vi "HandleError.vi"(8 "error in (no error)":errorcluster, 11 "Queue in":refnum<queue>) -> (0 "error out":errorcluster, 3 "queue out":refnum<queue>)   [LabVIEW 2019, in "AutoMode.lvlib"]
uses:
  AutoMode.lvlib
  Cluster - AutoModeMessage.ctl
  Enum - AutoModeState.ctl
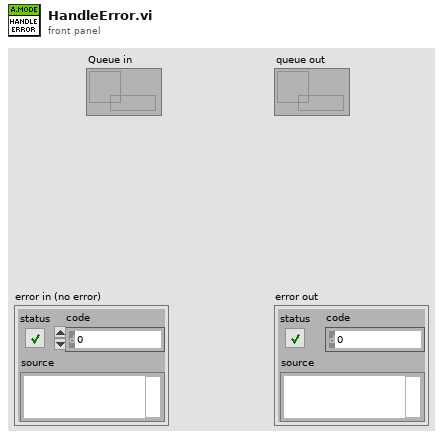
[diagram p1: front panel]
types:
  T1 = typedef "AutoMode.lvlib/Enum - AutoModeState.ctl" = enum16{"Initialize", "Idle", "UpdateConfig", "BroadcastSettings", "Start", "Winding", "WaitForWinding", "Unwind", "WaitForUnwind", "Stop", "Abort", "WriteDataToFile", "EventTriggered", "GenerateFilePath", "ZeroPosition", "GotoZero", "Error", "Exit"}
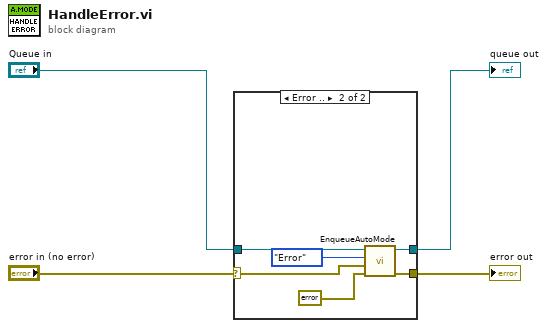
[diagram p0: block diagram]
diagram:
  n1 = case shown="Error .." "error in (no error)" {
    selector: "error in (no error)" -> [w5 w8]
    tunnel: [w5 w12] -> w4
    tunnel: "Queue in" -> [w6 w11]
    tunnel: [w6 w10] -> w1
    frame No Error {
    }
    frame Error {
      n2 = call "EnqueueAutoMode.vi"("error in (no error)"=errorcluster {"status"=FALSE, "code"=0, "source"=""}, "Data"=w8, "AutoState"=Enum_-_AutoModeState."Error" ("CycleTestState"), "Queue in"=w11) -> ("error out"=w12:errorcluster, "queue out"=w10:refnum<queue>)  [unwired: 6 in]
    }
  }
  "error out" <- w4
  "queue out" <- w1
